vi "get timing interval.vi"(8 "error in (no error)":errorcluster, 11 "ImagingModeSPIM in":refnum<class "ImagingModeSPIM.lvclass">) -> (0 "error out":errorcluster, 2 "dt":dbl, 3 "ImagingModeSPIM out":refnum<class "ImagingModeSPIM.lvclass">)   [LabVIEW 2012, in "ImagingModeSPIM.lvclass"]
uses:
  ImagingModeSPIM.lvclass
  ImagingModeSPIM.lvclass/ImagingModeSPIM.ctl
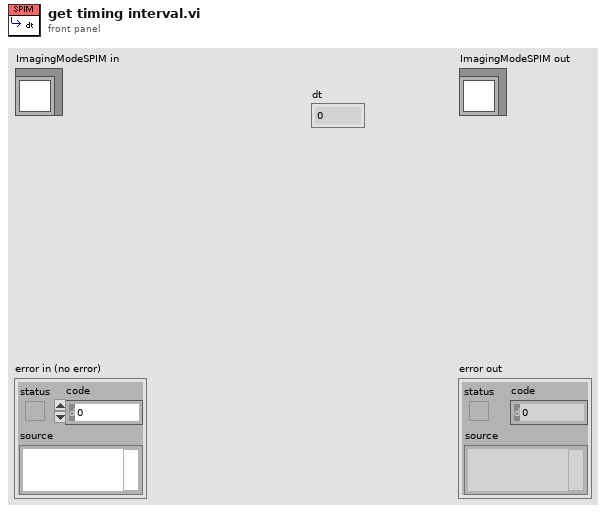
[diagram p1: front panel]
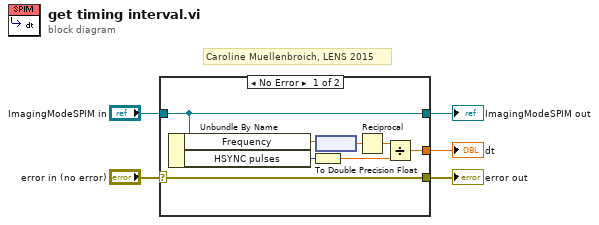
[diagram p0: block diagram]
diagram:
  # "Caroline Muellenbroich, LENS 2015"
  n1 = case shown="No Error" "error in (no error)" {
    selector: "error in (no error)" -> [w13 w15]
    tunnel: [w13 w15] -> w4
    tunnel: [w12 w14] -> w2
    tunnel: "ImagingModeSPIM in" -> [w12 w14]
    tunnel: [w6 _] -> w1
    frame No Error {
      n2 = Unbundle By Name(w12) -> ("Frequency"=w10:dbl[unit], "HSYNC pulses"=w9:i32)
      n3 = To Double Precision Float(number=w9) -> (double precision float=w7:dbl)
      n4 = node(w10) -> (w11:dbl)
      n5 = Reciprocal(x=w11) -> (1/x=w8:dbl)
      n6 = Divide(x=w8, y=w7) -> (x/y=w6:dbl)
    }
    frame Error {
    }
  }
  "error out" <- w4
  "ImagingModeSPIM out" <- w2
  "dt" <- w1
